vi "Get All Datatype groups.vi"(8 "error in (no error)":errorcluster, 11 "Channel group in":refnum<class "Channel group.lvclass">) -> (0 "error out":errorcluster, 1 "Datatype Groups":refnum<class "Datatype group.lvclass">[](array[class]), 2 "names":string[](array[string]), 3 "Channel group out":refnum<class "Channel group.lvclass">)   [LabVIEW 2016, in "FPGA RM Shared API.lvlib" / "Channel group.lvclass"]
uses:
  Channel group.lvclass
  Datatype Group/Datatype group.lvclass
  Channel group.lvclass/Channel group.ctl
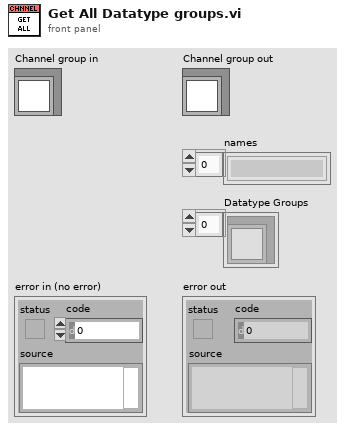
[diagram p1: front panel]
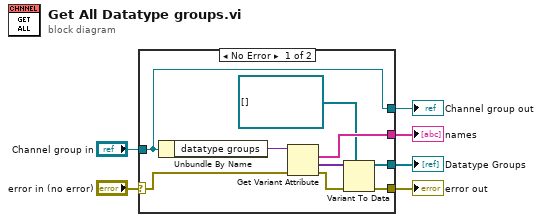
[diagram p0: block diagram]
diagram:
  n1 = case shown="No Error" "error in (no error)" {
    selector: "error in (no error)" -> [w8 w17]
    tunnel: [w11 w17] -> w5
    tunnel: [w15 w16] -> w3
    tunnel: "Channel group in" -> [w15 w16]
    tunnel: [w13 _] -> w2
    tunnel: [w9 _] -> w1
    frame No Error {
      n2 = Unbundle By Name(w15) -> ("datatype groups"=w14:variant)
      n3 = Get Variant Attribute(Variant=w14, error in=w8) -> (names=w13:string[], values=w12:variant[], error out=w7:errorcluster)  [unwired: 2 in, 1 out]
      n4 = Variant To Data(error in=w7, type=refnum<class "Datatype group.lvclass">[] [] ("Array"), Variant=w12) -> (data=w9:refnum<class "Datatype group.lvclass">[], error out=w11:errorcluster)
    }
    frame Error {
    }
  }
  "error out" <- w5
  "Channel group out" <- w3
  "names" <- w2
  "Datatype Groups" <- w1
